vi "Laser Power Control Messenger.vi"(0 "Wavelength (nm)":u16, 2 "Power Ctrl Actions":T2, 7 "Line On/Off":bool, 11 "Power":dbl) -> (4 "Wavelengths":u16[](array[numeric]), 15 "Power Status":T1[](array[typedef]))   [LabVIEW 2016]
uses:
  Laser Power Control Type Defs/Laser Power Ctrl Messenger Actions.ctl
  Laser Power Control Type Defs/Laser Power Ctrl Base Type.ctl
  Laser Power Control Type Defs/Laser Power Ctrl Notifier Type.ctl
  Laser Power Control Type Defs/Laser Power Ctrl Actions.ctl
panel:
  out "Error":errorcluster
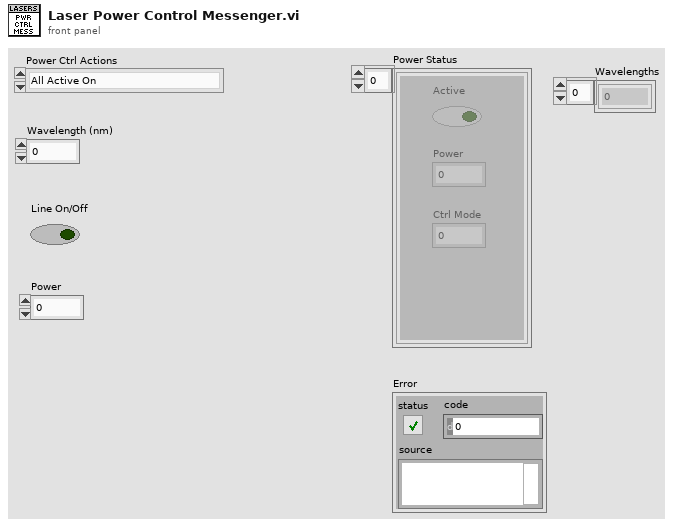
[diagram p1: front panel]
types:
  T1 = typedef "Laser Power Ctrl Base Type.ctl" = cluster{"Active":bool, "Power":dbl, "Ctrl Mode":u16}
  T2 = typedef "Laser Power Ctrl Messenger Actions.ctl" = enum16{"All Active On", "All Off", "Adjust Power", "Line On/Off", "Get Status"}
  T3 = typedef "Laser Power Ctrl Notifier Type.ctl" = cluster{"Actions":T4, "Wavelength":u16, "Wavelengths":u16[], "Power Ctrl":T1[]}
  T4 = typedef "Laser Power Ctrl Actions.ctl" = enum16{"Exit Loop", "Active", "Power Adj", "All Active On", "All Active Off", "Quit"}
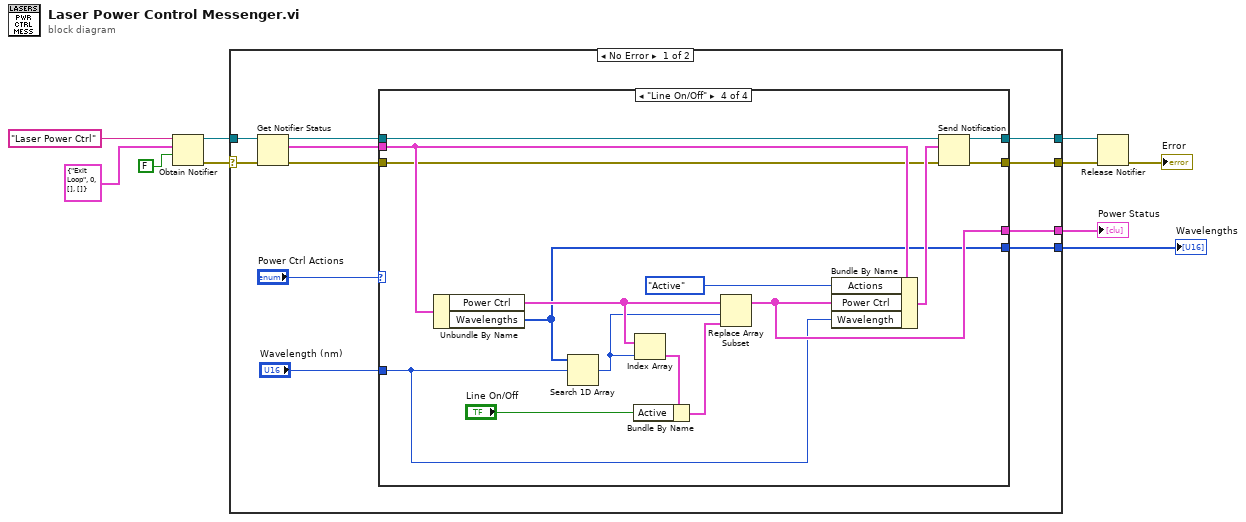
[diagram p0: block diagram]
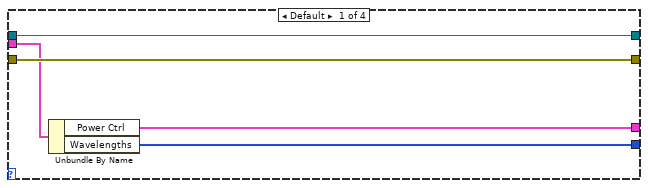
[diagram p2: hidden frame]
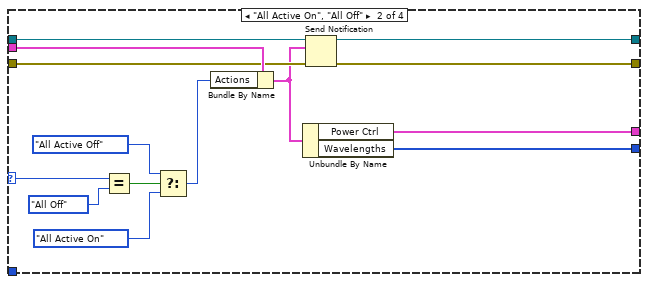
[diagram p3: hidden frame]
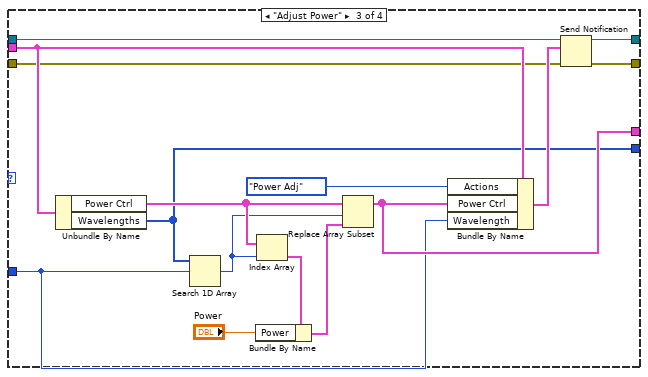
[diagram p4: hidden frame]
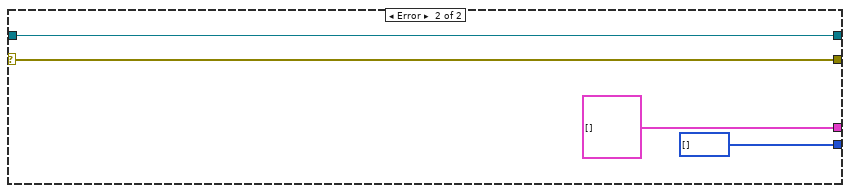
[diagram p5: hidden frame]
diagram:
  n1 = Obtain Notifier(name (unnamed)="Laser Power Ctrl", notification data type=T3 {"Actions"=enum."Exit Loop", "Wavelength"=0, "Wavelengths"=[], "Power Ctrl"=[]} ("Laser Power Ctrl Note Type"), create if not found? (T)=FALSE) -> (notifier out=w6:refnum<notifier>, error out=w7:errorcluster)  [unwired: 1 in, 1 out]
  n2 = case shown="No Error" w7 {
    selector: w7 -> [w21 w73]
    tunnel: w6 -> [w20 w74]
    tunnel: [w14 T1[] [] ("Power Ctrl")] -> w5
    tunnel: [w13 w74] -> w4
    tunnel: [w12 w73] -> w3
    tunnel: [w11 u16[] [] ("Wavelengths")] -> w1
    frame No Error {
      n3 = Get Notifier Status(notifier=w20, error in (no error)=w21) -> (notifier out=w19:refnum<notifier>, current notification=w17:T3, error out=w15:errorcluster)  [unwired: 2 out]
      n4 = case shown="\"Line On/Off\"" "Power Ctrl Actions" {
        selector: "Power Ctrl Actions" -> [_ w38 _ _]
        tunnel: w19 -> [w26 w40 w55 w70]
        tunnel: w17 -> [w24 w39 w48 w64]
        tunnel: "Wavelength (nm)" -> [_ _ w41 w56]
        tunnel: [w26 w32 w47 w62] -> w13
        tunnel: w15 -> [w25 w31 w45 w61]
        tunnel: [w23 w28 w43 w59] -> w14
        tunnel: [w25 w30 w44 w58] -> w12
        tunnel: [w22 w27 w42 w57] -> w11
        frame Default {
          n5 = Unbundle By Name(w24) -> ("Power Ctrl"=w23:T1[], "Wavelengths"=w22:u16[])
        }
        frame "All Active On", "All Off" {
          n6 = Equal?(x=w38, y=Laser_Power_Ctrl_Messenger_Actions."All Off") -> (x = y?=w36:bool)
          n7 = Select(t=Laser_Power_Ctrl_Actions."All Active Off" ("Actions"), s=w36, f=Laser_Power_Ctrl_Actions."All Active On" ("Actions")) -> (s? t:f=w33:T4)
          n8 = Bundle By Name(cluster=w39, "Actions"=w33) -> (w29:T3)
          n9 = Unbundle By Name(w29) -> ("Power Ctrl"=w28:T1[], "Wavelengths"=w27:u16[])
          n10 = Send Notification(notification=w29, notifier=w40, error in (no error)=w31) -> (notifier out=w32:refnum<notifier>, error out=w30:errorcluster)
        }
        frame "Adjust Power" {
          n11 = Unbundle By Name(w48) -> ("Power Ctrl"=w52:T1[], "Wavelengths"=w42:u16[])
          n12 = Search 1D Array(1D array=w42, element=w41) -> (index of element=w50:i32)  [unwired: 1 in]
          n13 = Index Array(array=w52, index=w50) -> (element=w54:T1)
          n14 = Bundle By Name(cluster=w54, "Power"="Power") -> (w51:T1)
          n15 = Replace Array Subset(array=w52, new element=w51, index=w50) -> (w43:T1[])
          n16 = Bundle By Name(cluster=w48, "Actions"=Laser_Power_Ctrl_Actions."Power Adj", "Power Ctrl"=w43, "Wavelength"=w41) -> (w49:T3)
          n17 = Send Notification(notification=w49, notifier=w55, error in (no error)=w45) -> (notifier out=w47:refnum<notifier>, error out=w44:errorcluster)
        }
        frame "Line On/Off" {
          n18 = Unbundle By Name(w64) -> ("Power Ctrl"=w68:T1[], "Wavelengths"=w57:u16[])
          n19 = Search 1D Array(1D array=w57, element=w56) -> (index of element=w66:i32)  [unwired: 1 in]
          n20 = Index Array(array=w68, index=w66) -> (element=w69:T1)
          n21 = Bundle By Name(cluster=w69, "Active"="Line On/Off") -> (w67:T1)
          n22 = Replace Array Subset(array=w68, new element=w67, index=w66) -> (w59:T1[])
          n23 = Bundle By Name(cluster=w64, "Actions"=Laser_Power_Ctrl_Actions."Active", "Power Ctrl"=w59, "Wavelength"=w56) -> (w65:T3)
          n24 = Send Notification(notification=w65, notifier=w70, error in (no error)=w61) -> (notifier out=w62:refnum<notifier>, error out=w58:errorcluster)
        }
      }
    }
    frame Error {
    }
  }
  "Power Status" <- w5
  "Wavelengths" <- w1
  n25 = Release Notifier(notifier=w4, error in (no error)=w3) -> (error out=→"Error":errorcluster)  [unwired: 1 in, 2 out]
